vi "Update.vi"(8 "error in (no error)":errorcluster, 10 "Message in":refnum<class "UpdateMessage.lvclass">, 11 "Autofocus in":refnum<class "Autofocus.lvclass">) -> (0 "error out":errorcluster, 3 "Autofocus out":refnum<class "Autofocus.lvclass">)   [LabVIEW 2012, in "Autofocus.lvclass"]
doc: "The update method processes the command 'update'. \n\nThe command 'update' is used for receiving new values to be set to the private data of the class. This could be seen as a public set method for setting new parameters to the private class data."
uses:
  Autofocus.lvclass
  <vilib>/Distrio/Murmex/UpdateMessage/UpdateMessage.lvclass
  Sharpness Measure.ctl
  Autofocus.lvclass/Autofocus.ctl
  ROI size.ctl
  Search algorithm.ctl
  <vilib>/Distrio/Murmex/Murmex/Murmex.lvclass
panel:
  # "This method is called when the UPDATE\ntrigger is sent. \n\nOverride this method when your component needs to\nrespond to this trigger. \n\nCall parent for proper implementation"
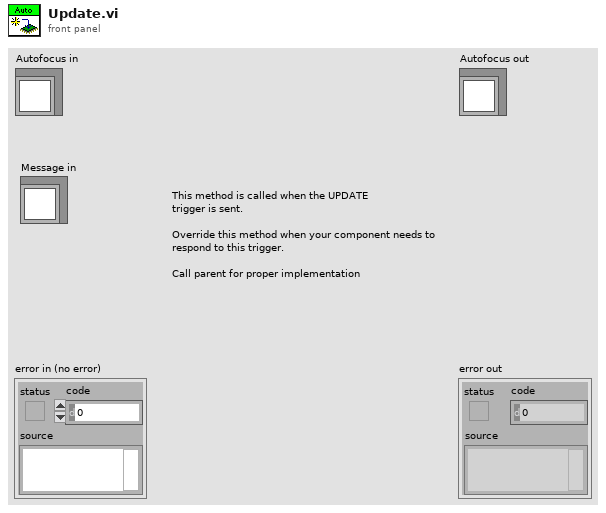
[diagram p1: front panel]
types:
  T1 = typedef "Autofocus.lvclass/Sharpness Measure.ctl" = enum16{"Vol4", "Gradient Square"}
  T2 = typedef "Autofocus.lvclass/Search algorithm.ctl" = enum16{"Hill Climbing"}
  T3 = typedef "Autofocus.lvclass/ROI size.ctl" = u16
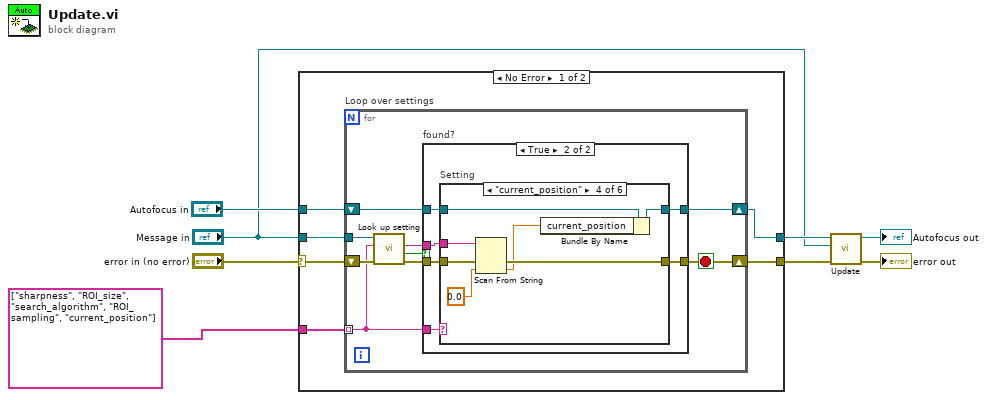
[diagram p0: block diagram]
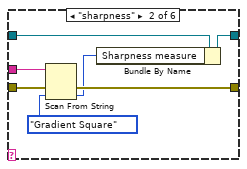
[diagram p4: hidden frame]
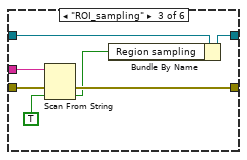
[diagram p5: hidden frame]
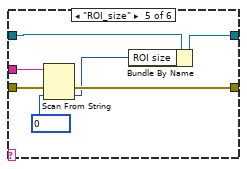
[diagram p6: hidden frame]
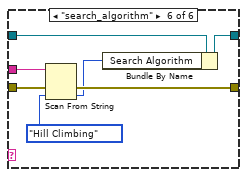
[diagram p7: hidden frame]
diagram:
  n1 = case shown="No Error" "error in (no error)" {
    selector: "error in (no error)" -> [w14 w70]
    tunnel: "Autofocus in" -> [w10 w69]
    tunnel: [w13 w70] -> w5
    tunnel: string[] ["sharpness", "ROI_size", "search_algorithm", "ROI_sampling", "current_position"] -> [w12 _]
    tunnel: "Message in" -> [w11 _]
    tunnel: [w9 w69] -> w3
    frame No Error {
      n2 = for "Loop over settings" {
        shift-right: [w17] -> w13
        shift-left: w14 -> [w23]
        shift-right: [w18] -> w9
        shift-left: w10 -> [w21]
        tunnel: w12 -> [w16] mode=indexing
        tunnel: w11 -> [w15]
        stop <- w17 stop-if-true
        n3 = call <vilib>:"Look up setting.vi"("error in (no error)"=w23, "tag name"=w16, "UpdateMessage in"=w15) -> ("error out"=w19:errorcluster, "found?"=w22:bool, "value"=w20:string)  [unwired: 5 in, 1 out]
        n4 = case "found?" shown="True" w22 {
          tunnel: w21 -> [w25 w29]
          tunnel: w20 -> [_ w30]
          tunnel: w19 -> [w24 w28]
          tunnel: w16 -> [_ w31]
          tunnel: [w25 w27] -> w18
          tunnel: [w24 w26] -> w17
          frame False {
          }
          frame True {
            n5 = case "Setting" shown="\"current_position\"" w31 {
              tunnel: w30 -> [_ w39 w45 w52 w55 w66]
              tunnel: w29 -> [w33 w38 w43 w51 w58 w64]
              tunnel: w28 -> [w32 w40 w47 w54 w61 w68]
              tunnel: [w33 w37 w42 w50 w56 w63] -> w27
              tunnel: [w32 w36 w46 w53 w60 w67] -> w26
              frame Default {
              }
              frame "sharpness" {
                n6 = Scan From String(input string=w39, error in=w40, default 1=Sharpness_Measure."Gradient Square" ("Sharpness measure")) -> (error out=w36:errorcluster, output 1=w34:T1)  [unwired: 2 in, 2 out]
                n7 = Bundle By Name(cluster=w38, "Sharpness measure"=w34) -> (w37:refnum<class "Autofocus.lvclass">)
              }
              frame "ROI_sampling" {
                n8 = Scan From String(input string=w45, error in=w47, default 1=TRUE) -> (error out=w46:errorcluster, output 1=w41:bool)  [unwired: 2 in, 2 out]
                n9 = Bundle By Name(cluster=w43, "Region sampling"=w41) -> (w42:refnum<class "Autofocus.lvclass">)
              }
              frame "current_position" {
                n10 = Scan From String(input string=w52, error in=w54, default 1=0.0 ("Settings cluster.current_position")) -> (error out=w53:errorcluster, output 1=w48:dbl)  [unwired: 2 in, 2 out]
                n11 = Bundle By Name(cluster=w51, "current_position"=w48) -> (w50:refnum<class "Autofocus.lvclass">)
              }
              frame "ROI_size" {
                w59 = T3 0 items=["50x50"=50, "100x100"=100, "250x250"=250] ("ROI size")
                n12 = Scan From String(input string=w55, error in=w61, default 1=w59) -> (error out=w60:errorcluster, output 1=w57:T3)  [unwired: 2 in, 2 out]
                n13 = Bundle By Name(cluster=w58, "ROI size"=w57) -> (w56:refnum<class "Autofocus.lvclass">)
              }
              frame "search_algorithm" {
                n14 = Scan From String(input string=w66, error in=w68, default 1=Search_algorithm."Hill Climbing" ("Search Algorithm")) -> (error out=w67:errorcluster, output 1=w62:T2)  [unwired: 2 in, 2 out]
                n15 = Bundle By Name(cluster=w64, "Search Algorithm"=w62) -> (w63:refnum<class "Autofocus.lvclass">)
              }
            }
          }
        }
      }
    }
    frame Error {
    }
  }
  n16 = call-parent "Update.vi"("error in (no error)"=w5, "Message in"="Message in", "Murmex in"=w3) -> ("error out"=→"error out":errorcluster, "Murmex out"=→"Autofocus out":refnum<class "Autofocus.lvclass">)  [unwired: 7 in]
